vi "IsUDCInstalled.vi"(0 "Error Out":errorcluster) -> (3 "Installed?":bool, 8 "Error Out":errorcluster)   [LabVIEW 2017, in "niceiplib.lvlib"]
doc: "UDC_SYMBOLS int IsUDCInstalled();\n\nThis vi returns true if UDC/CEIP is installed on this system. Returns false if UDC/CEIP is not installed."
uses:
  <vilib>/UDC/niceiplib.lvlib
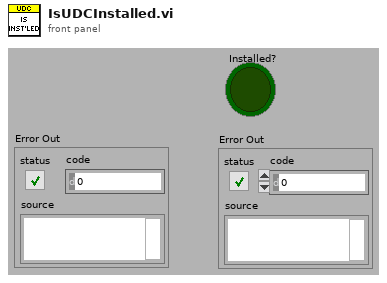
[diagram p1: front panel]
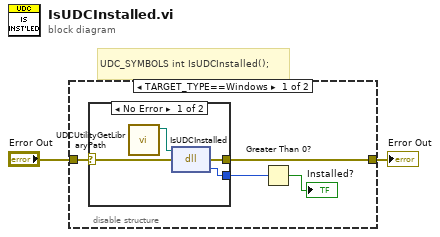
[diagram p0: block diagram]
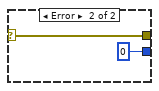
[diagram p2: hidden frame]
diagram:
  # "UDC_SYMBOLS int IsUDCInstalled();"
  n1 = disable-structure shown="TARGET_TYPE==Windows" {
    disable-tunnel: [w5 w13] -> w2
    disable-tunnel: "Error Out" -> [w4 w13]
    frame condition #0 (active) {
      n2 = case shown="No Error" w4 {
        selector: w4 -> [w8 w12]
        tunnel: [w10 0 ("return type")] -> w6
        tunnel: [w9 w12] -> w5
        frame No Error {
          n3 = call <vilib>:"UDCUtilityGetLibraryPath.vi"() -> ("Library Path"=w7:path)  [unwired: 11 in]
          n4 = dll-call lib="C:/2013LabVIEWCode/dist/vi.lib/UDC/niceiplib.*" fn="IsUDCInstalled"(path in=w7, error in=w8) -> (error out=w9:errorcluster, "return type"=w10:i32)  [unwired: 1 in, 1 out]
        }
        frame Error {
        }
      }
      n5 = Greater Than 0?(x=w6) -> (x > 0?=→"Installed?":bool)
    }
    frame condition #1 {
    }
  }
  "Error Out" <- w2
